vi "AR-DI-close.vi"(8 "error in (no error)":errorcluster, 11 "DI task in":refnum<k21>) -> (0 "error out":errorcluster)   [LabVIEW 2021]
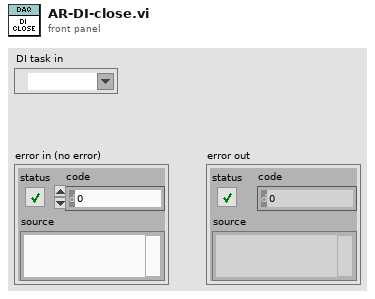
[diagram p1: front panel]
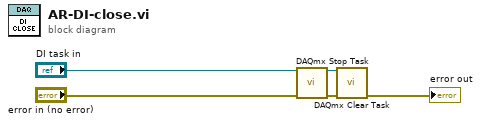
[diagram p0: block diagram]
diagram:
  n1 = call <vilib>:"DAQmx Stop Task.vi"("task/channels in"="DI task in", "error in"="error in (no error)") -> ("task out"=w3:refnum<k21>, "error out"=w4:errorcluster)  [unwired: 12 in]
  n2 = call <vilib>:"DAQmx Clear Task.vi"("task in"=w3, "error in"=w4) -> ("error out"=→"error out":errorcluster)  [unwired: 13 in]
